vi "Convert ASCII to Unicode.vi"() -> ()   [LabVIEW 2009]
panel:
  out "Unicode displayed on an ASCII indicator":string
  out "ASCII (hex)":string
  out "Unicode (hex)":string
  out "ASCII (hex)":string
  out "ASCII":string
  out "Unicode":string
  in  "ASCII":string="Hello World"
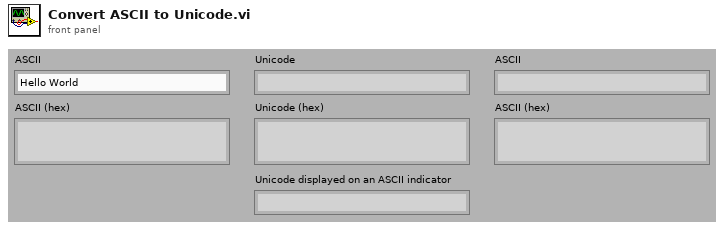
[diagram p1: front panel]
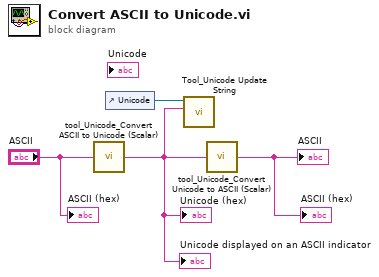
[diagram p0: block diagram]
diagram:
  n1 = call "tool_Unicode_Convert ASCII to Unicode (Scalar).vi"("ASCII"="ASCII") -> ("Unicode"=w1:string)  [unwired: 4 in]
  "Unicode (hex)" <- w1
  "Unicode displayed on an ASCII indicator" <- w1
  n2 = control-ref of="Unicode"() -> (w2:refnum<vi>)
  n3 = call "Tool_Unicode Update String.vi"("String Value"=w1, "String Control Reference"=w2) -> ()  [unwired: 6 in, 2 out]
  n4 = call "tool_Unicode_Convert Unicode to ASCII (Scalar).vi"("Unicode"=w1) -> ("ASCII"=→"ASCII" →"ASCII (hex)":string)  [unwired: 4 in]
  "ASCII (hex)" <- "ASCII"
